vi "DSF.Engine.Plugin.Initialize_v1.vi"(7 "Device Ref in":T1=18446744073709551615 format="%.0x", 8 "error in (no error)":errorcluster, 10 "Configuration":refnum<class "DSF.Shared.Configuration.Plugin.lvclass">, 11 "Plugin type":refnum<class "Plugin.lvclass">) -> (0 "error out":errorcluster, 3 "Plugin out":refnum<class "Plugin.lvclass">)   [LabVIEW 2017, in "DSF.Engine.lvlib" / "Plugin.lvclass"]
uses:
  Plugin.lvclass
  Shared/Classes/Plugin/DSF.Shared.Configuration.Plugin.lvclass
  Transfer/DSF.Engine.Transfer Group.lvclass
  Transfer/DSF.Engine.Transfer.lvclass
  Interface/DSF.Engine.Interface.Plugin.lvclass
  <vilib>/NI Veristand/Custom Device API/Custom Device Item Ref.ctl
  <vilib>/NI Veristand/Custom Device API/Custom Device API.lvlib
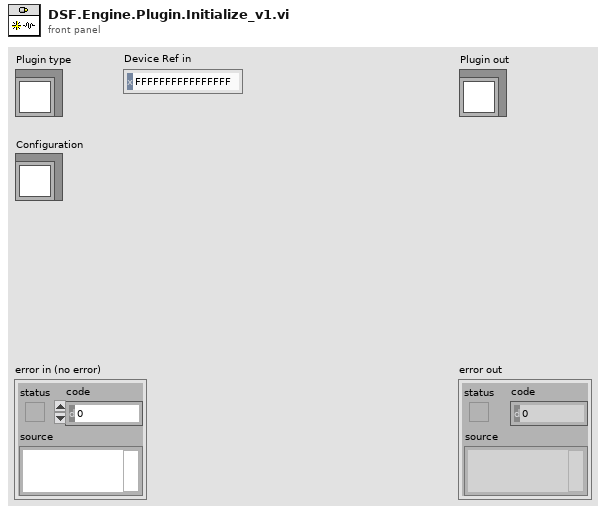
[diagram p1: front panel]
types:
  T1 = typedef "Custom Device API.lvlib/Custom Device Item Ref.ctl" = u64
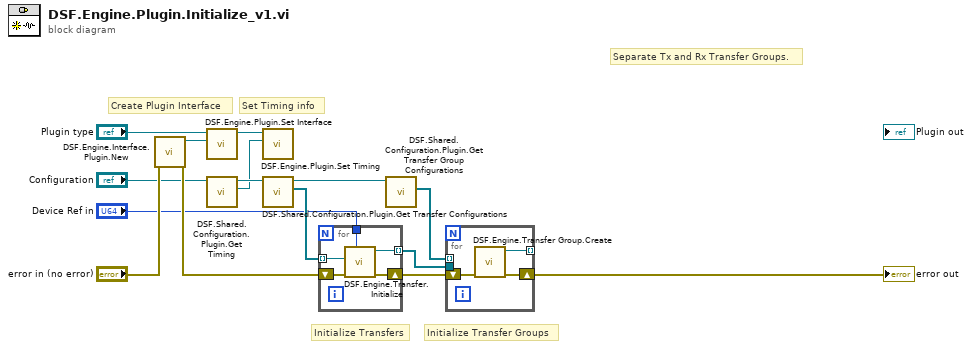
[diagram p0: block diagram]
diagram:
  # "Separate Tx and Rx Transfer Groups."
  # "Set Timing info"
  # "Create Plugin Interface"
  # "Initialize Transfer Groups"
  # "Initialize Transfers"
  n1 = call "DSF.Engine.Interface.Plugin.New.vi"("error in (no error)"="error in (no error)") -> ("error out"=w3:errorcluster, "Plugin Interface"=w5:refnum<class "DSF.Engine.Interface.Plugin.lvclass">)  [unwired: 9 in]
  n2 = call "DSF.Engine.Plugin.Set Interface.vi"("Interface"=w5, "Plugin in"="Plugin type") -> ("Plugin out"=w15:refnum<class "Plugin.lvclass">)  [unwired: 9 in]
  n3 = call "DSF.Shared.Configuration.Plugin.Get Timing.vi"("Plugin Configuration in"="Configuration") -> ("Timing"=w7:refnum<class "DSF.Shared.Timing.lvclass">, "Plugin Configuration out"=w14:refnum<class "DSF.Shared.Configuration.Plugin.lvclass">)  [unwired: 9 in]
  n4 = call "DSF.Engine.Plugin.Set Timing.vi"("Timing"=w7, "Plugin in"=w15) -> ()  [unwired: 9 in, 1 out]
  n5 = call "DSF.Shared.Configuration.Plugin.Get Transfer Configurations.vi"("Plugin Configuration in"=w14) -> ("Transfer Configurations"=w13:refnum<class "DSF.Shared.Configuration.Transfer.lvclass">[], "Plugin Configuration out"=w11:refnum<class "DSF.Shared.Configuration.Plugin.lvclass">)  [unwired: 9 in]
  n6 = for {
    tunnel: w13 -> [w20] mode=indexing
    tunnel: [w19] -> w9 mode=indexing
    tunnel: "Device Ref in" -> [w18]
    shift-right: [w17] -> w10
    shift-left: w3 -> [w16]
    n7 = call "DSF.Engine.Transfer.Initialize.vi"("Device Ref in"=w18, "error in (no error)"=w16, "Configuration"=w20) -> ("error out"=w17:errorcluster, "Transfer out"=w19:refnum<class "DSF.Engine.Transfer.lvclass">)  [unwired: 7 in]
  }
  n8 = call "DSF.Shared.Configuration.Plugin.Get Transfer Group Configurations.vi"("Plugin Configuration in"=w11) -> ("Transfer Group Configurations"=w12:refnum<class "DSF.Shared.Configuration.Transfer Group.lvclass">[])  [unwired: 9 in, 1 out]
  n9 = for {
    tunnel: w9 -> [_]
    tunnel: w12 -> [_] mode=indexing
    tunnel: [w21] -> _ mode=indexing
    shift-right: [w23] -> w8
    shift-left: w10 -> [w22]
    n10 = call "DSF.Engine.Transfer Group.Create.vi"("error in (no error)"=w22) -> ("error out"=w23:errorcluster, "Transfer Group out"=w21:refnum<class "DSF.Engine.Transfer Group.lvclass">)  [unwired: 9 in]
  }
  "error out" <- w8
